vi "Migrate InstrumentStudio Plug-in.vi"() -> ()   [LabVIEW 2021]
uses:
  _Measurement Migrator/Migrator/Queue Driver/controls/Queue Operations.ctl
  _Measurement Migrator/Migrator/Migration Logic/controls/Multiple Migration/Multiple Migration Data Holder.ctl
  <vilib>/Utility/sysdir.llb/System Directory Type.ctl
  <vilib>/Utility/miscctls.llb/LVRowAndColumnUnsignedTypeDef.ctl
  <vilib>/Utility/miscctls.llb/LVRowAndColumnTypeDef.ctl
  _Measurement Migrator/Migrator/Migrator Reusables/controls/Dictionary States.ctl
  <vilib>/Utility/cursorutil.llb/Set Cursor (Icon Pict).vi
  _Measurement Migrator/Migrator/Queue Driver/Queue Driver.lvlib
  _Measurement Migrator/Migrator/Migration Logic/Migrator.lvlib
  _Measurement Migrator/Migrator/Path Functions/Path Functions.lvlib
  _Measurement Migrator/Migrator/Multiple Migrator/Multiple Migrator.lvlib
  _Measurement Migrator/Migrator/Migrator Reusables/Migrator Reusables.lvlib
  _Measurement Migrator/Migrator/G Plug-in Migrator/G Plug-in Migrator.lvlib
panel:
  out "error out":errorcluster
  in  "Tab Control":T1(tab)
  in  "Info":string
  in  "Select Measurement":path
  out "Warning":bool=TRUE caption="Warning:\nSelected folder contains invalid folder/file names"
  in  "Populate measurements":bool
  in  "Select Project":path
  in  "Select all":bool
  in  "Back to Home":bool
  in  "List Plug-ins":bool
  in  "Select Measurements":string(tree)
  out "Selection warning":string="Atleast one measurement should be selected"
  out "Plug-in info":string="* Rename the Plug-in if required"
  out "Plug-in warning":string="Warning:\n1. Measurement plug-in name must be unique \n2. Plugin name cannot contain any of the following characters:\n         \\ / : * ? \" < > |"
  in  "Start Migration":bool
  in  "Back to Select":bool
  in  "List of Selected Measurements":i32(listbox)
  in  "Measurement Count":i32(slide)=6 caption="Migrating 2 of 2 measurement(s)" scale=0.0..100.0
  in  "Progress":i32(slide)=9 caption="Saving the project files..." scale=0.0..15.0
  in  "Review":bool
  in  "Migration Status":i32(listbox)
  in  "Back to Status":bool
  in  "Select Plug-in":string(combo) caption="Select G plug-in to review"
  in  "Start Next":bool
  out "Launch Gplugin":string
  out "Launch VI":string
  # "* Project in which the measurement plug-in will be created"
  # "* Select a measurement vi or a folder containing measurements"
  # ".lvproj"
  # "Select the measurements to migrate"
  # "Review the G Plug-in:\n1. Review the Main VI. Click here to launch.\n2. Review the G plug-in data file. Click here to launch."
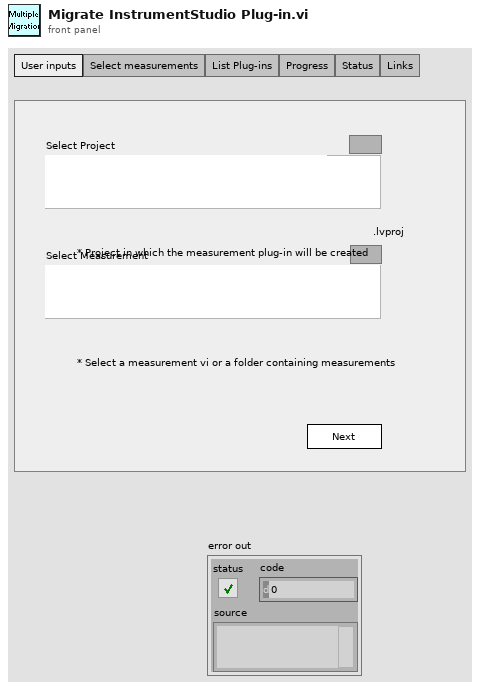
[diagram p1: front panel]
types:
  T1 = enum32{"User inputs", "Select measurements", "List Plug-ins", "Progress", "Status", "Links"}
  T2 = typedef "Queue Driver.lvlib/Queue Operations.ctl" = enum16{"Create Q", "Enqueue", "Enqueue N", "Dequeue", "Flush", "Release"}
  T3 = typedef "Migrator.lvlib/Multiple Migration Data Holder.ctl" = cluster{"Tree Reference":refnum<vi>, "LabVIEW Version":string, "Project path":path, "Create new project?":bool, "Measurement file/folder path":path, "Measurement folder selected?":bool, "Project warning":string, "Measurement warning":string, "Next clicked?":bool, "Measurement path changed?":bool, "Select all":bool, "Measurement folder Tags":string[], "Measurement file Tags":string[], "Selected cell Tag":string, "Measurement Plug-ins":string[][], "Measurement File Paths":path[], "Plugin Migration Value":i32, "Migration Count":i32, "Instrument containing subVIs":path[][], "Progress per measurement":i32, "Measurement Progress":i32, "Migration Status":string[][], "Selected Measurement":string[], "G plugin Path":path[], "Plugin data file":path[], "Index":i32}
  T4 = enum8{"Enabled", "Disabled", "Disabled and Grayed Out"}
  T5 = typedef "LVRowAndColumnUnsignedTypeDef.ctl" = cluster{"Row":u32, "Column":u32}
  T6 = typedef "LVRowAndColumnTypeDef.ctl" = cluster{"Row":i32, "Column":i32}
  T7 = typedef "Migrator Reusables.lvlib/Dictionary States.ctl" = enum16{"Set", "Get", "Delete", "Delete All"}
  T8 = typedef "System Directory Type.ctl" = i32
  T9 = typedef "LVPoint32TypeDef.ctl" = cluster{"Horizontal":i32, "Vertical":i32}
  T10 = typedef "Migrator.lvlib/Tree Items.ctl" = cluster{"Item name":string, "Indent":i32, "Tag":string}
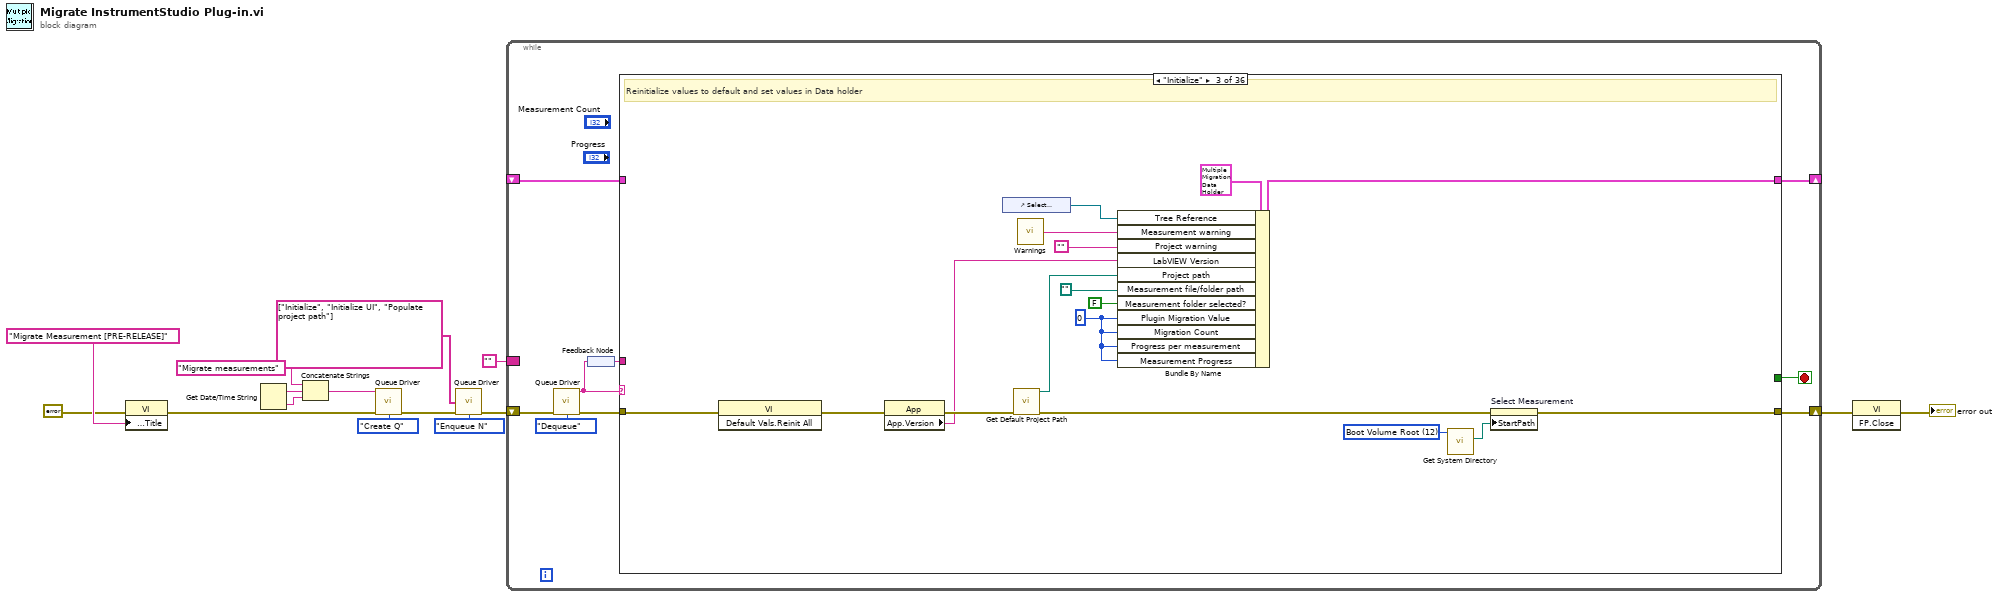
[diagram p0: block diagram]
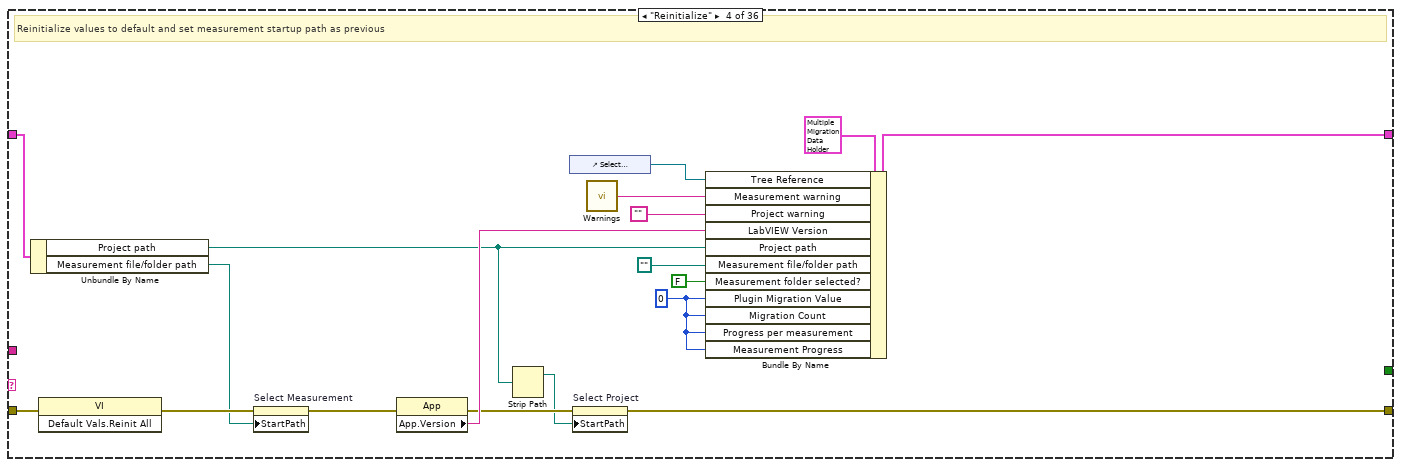
[diagram p4: hidden frame]
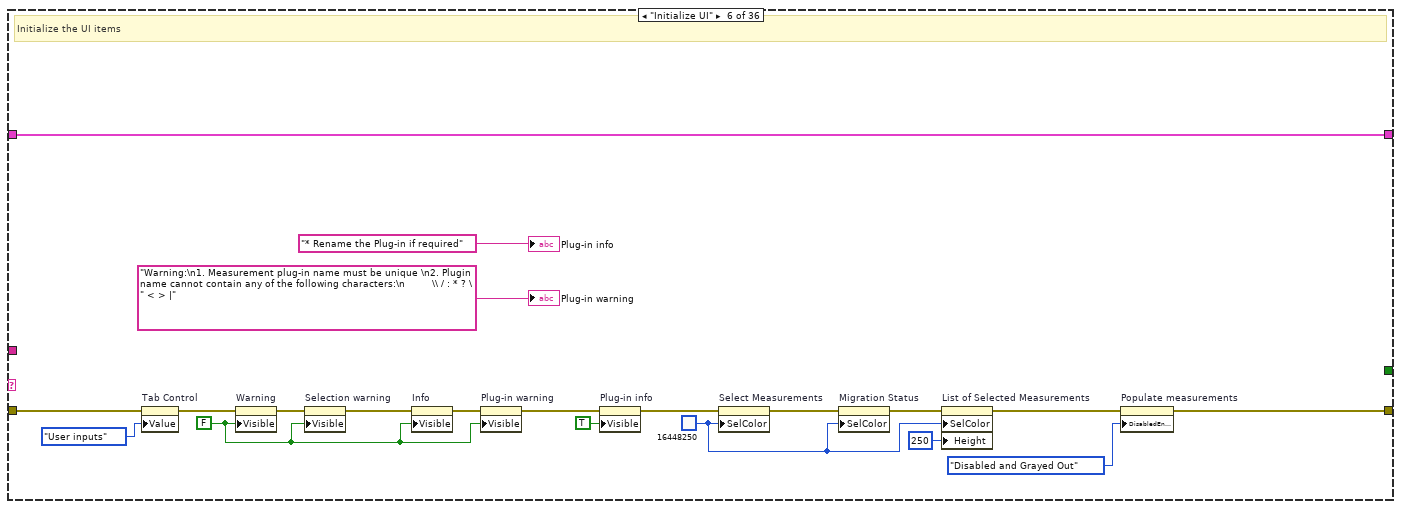
[diagram p6: hidden frame]
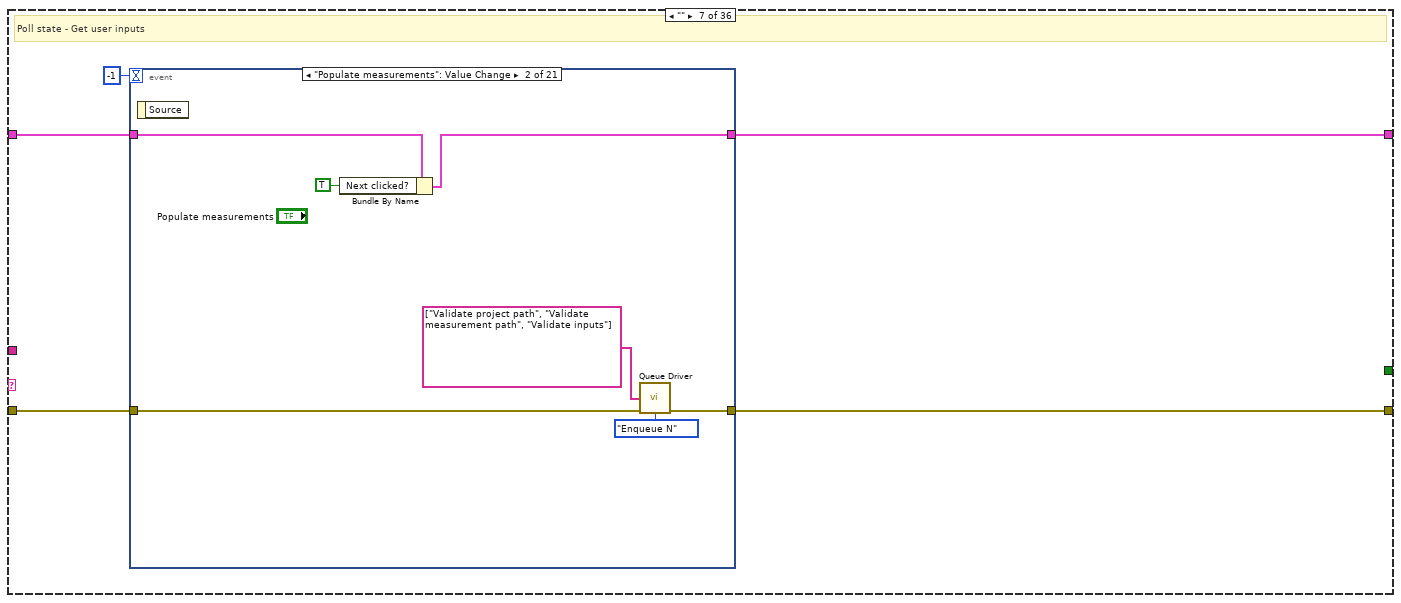
[diagram p7: hidden frame]
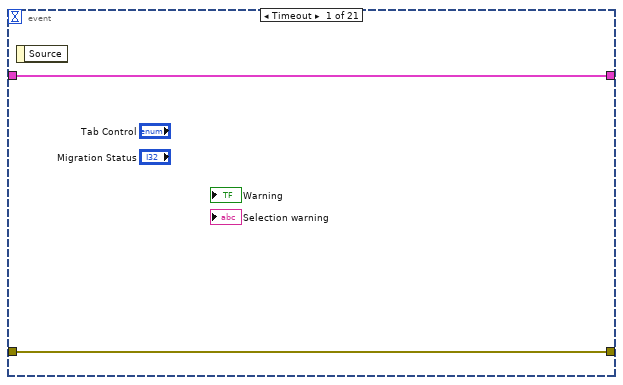
[diagram p8: hidden frame]
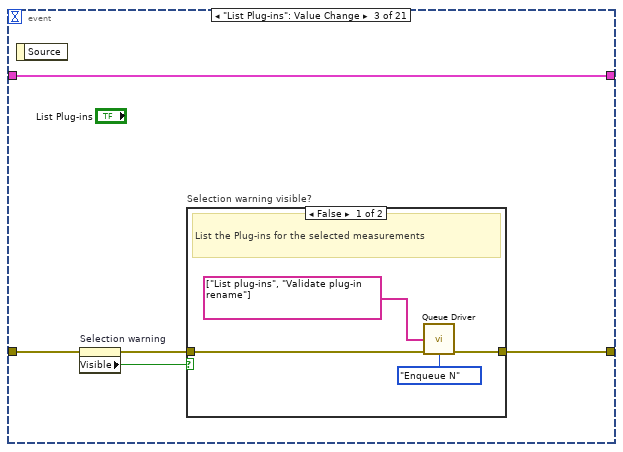
[diagram p9: hidden frame]
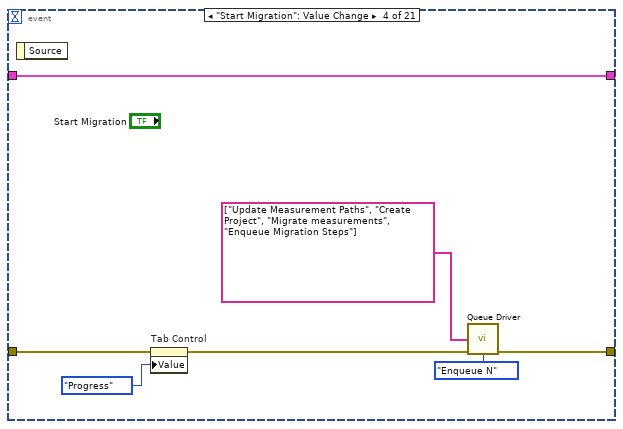
[diagram p11: hidden frame]
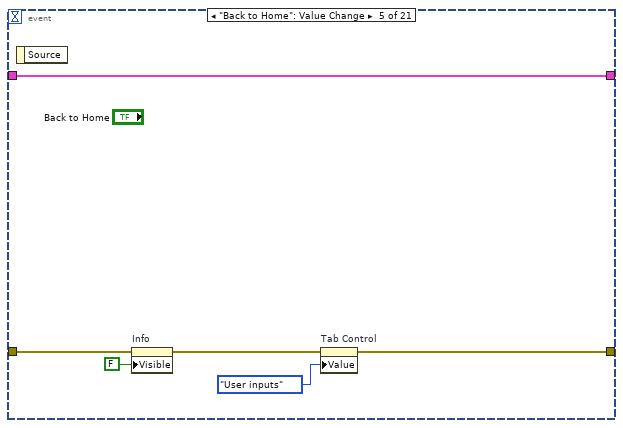
[diagram p12: hidden frame]
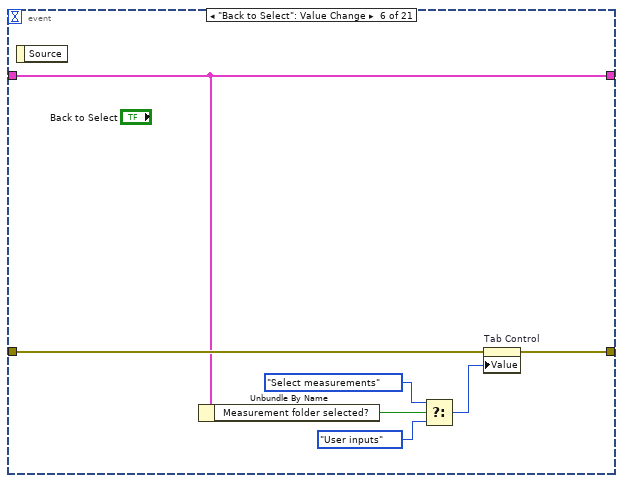
[diagram p13: hidden frame]
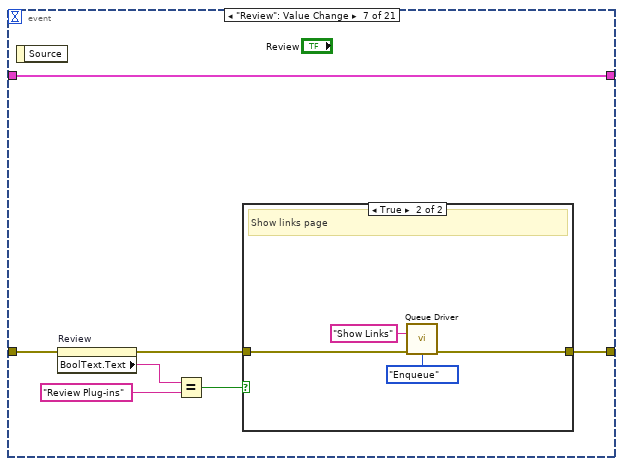
[diagram p14: hidden frame]
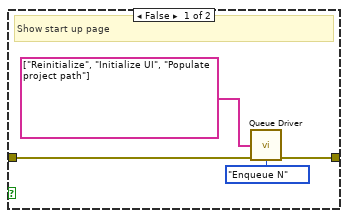
[diagram p15: hidden frame]
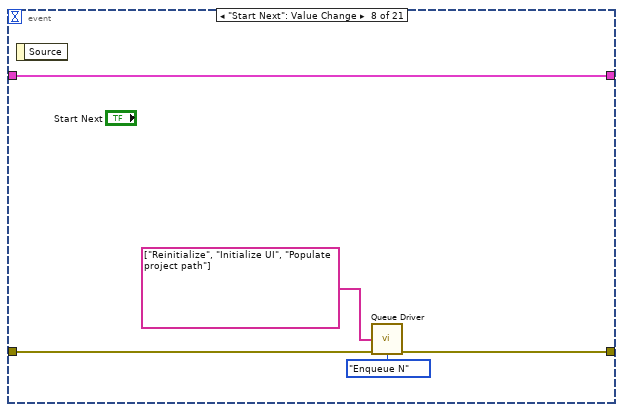
[diagram p16: hidden frame]
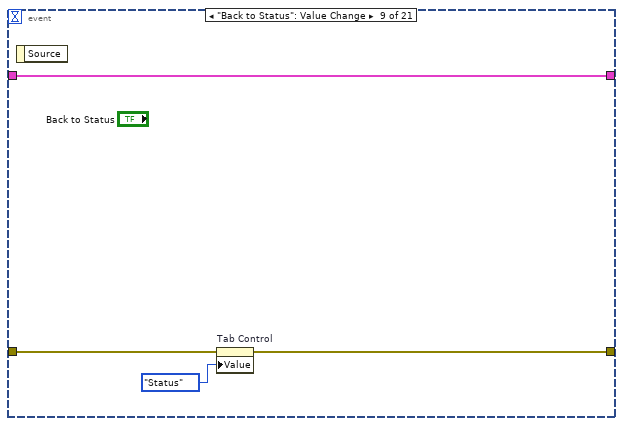
[diagram p17: hidden frame]
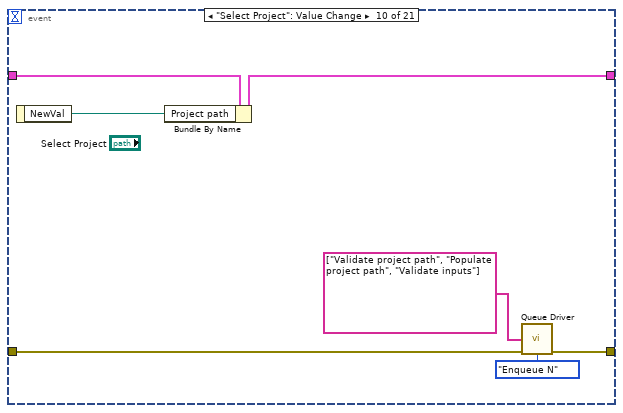
[diagram p18: hidden frame]
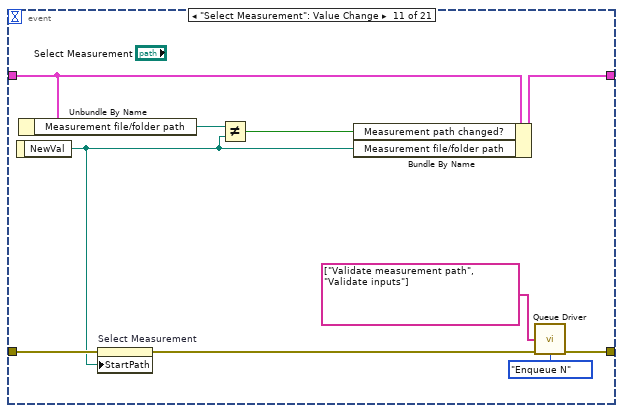
[diagram p19: hidden frame]
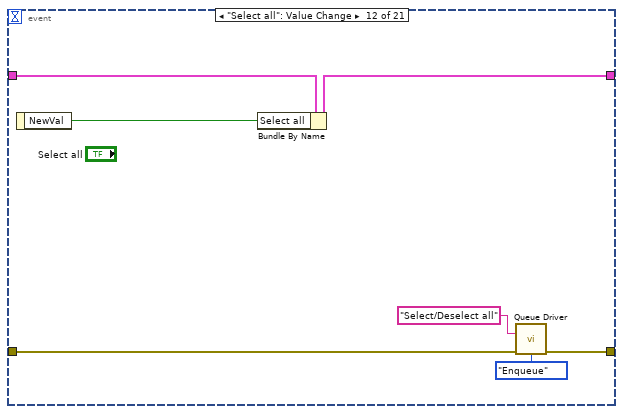
[diagram p20: hidden frame]
diagram:
  n1 = property class="VI"(error in=errorcluster {"status"=FALSE, "code"=0, "source"=""} ("error in (no error)"), "Front Panel.Title"="Migrate Measurement [PRE-RELEASE]" ("Front Panel Window:Title")) -> (error out=w1:errorcluster)  [unwired: 1 in, 1 out]
  n2 = Get Date/Time String() -> (date string=w12:string, time string=w11:string)  [unwired: 3 in]
  n3 = Concatenate Strings("Migrate measurements" ("string"), w12, w11) -> (w7:string)
  n4 = call "Queue Driver.vi"("Name"=w7, "error in (no error)"=w1, "Q Operations"=Queue_Operations."Create Q") -> ("error out"=w15:errorcluster)  [unwired: 11 in, 1 out]
  n5 = call "Queue Driver.vi"("States[]"=string[] ["Initialize", "Initialize UI", "Populate project path"], "error in (no error)"=w15, "Q Operations"=Queue_Operations."Enqueue N") -> ("error out"=w10:errorcluster)  [unwired: 11 in, 1 out]
  n6 = while {
    shift-right: [w23] -> w6
    shift-left: w10 -> [w24]
    shift-right: [w20] -> _
    shift-left: _ -> [w19]
    border: "" -> [_]
    stop <- w18 stop-if-true
    n7 = call "Queue Driver.vi"("error in (no error)"=w24, "Q Operations"=Queue_Operations."Dequeue") -> ("Dequeued State"=w17:string, "error out"=w22:errorcluster)  [unwired: 12 in]
    n8 = feedback #1() -> (w16:string)
    n9 = feedback-in #1(w17) -> ()
    n10 = case shown="\"Initialize\"" w17 {
      tunnel: w22 -> [w25 w28 w45 w63 w65 w85 w90 w258 w270 w281 w300 w324 w369 w386 w439 w464 w485 w511 w547 w557 w564 w584 w594 w613 w630 w664 w673 w679 w701 w722 w734 w777 w786 w795 w816 w828]
      tunnel: [w25 w28 w34 w48 w65 w76 w89 w260 w270 w273 w299 w323 w369 w381 w427 w447 w472 w510 w537 w557 w559 w581 w597 w612 w629 w650 w674 w683 w705 w722 w733 w774 w786 w792 w816 w818] -> w23
      tunnel: [w26 w27 w44 w62 w64 w81 w86 w259 w271 w276 w293 w311 w370 w387 w430 w462 w469 w508 w542 w556 w576 w592 w606 w616 w649 w651 w677 w684 w706 w723 w738 w769 w787 w797 w817 w826] -> w20
      tunnel: w19 -> [w26 w27 _ w51 w64 w81 w87 w259 w271 w277 w295 w322 w370 w388 w431 w463 w470 w509 w543 w556 w577 w592 w605 w616 w649 w653 w677 w685 w707 w723 w739 w776 w787 w797 w817 w826]
      tunnel: [_ _ _ _ _ _ _ _ _ _ _ _ _ _ _ _ _ _ _ _ _ _ _ _ _ _ _ _ _ _ _ _ _ _ _ TRUE] -> w18
      tunnel: w16 -> [_ _ _ _ _ _ _ _ _ _ _ _ _ _ _ _ _ _ _ _ _ _ _ _ _ _ _ _ _ _ _ _ _ w788 _ _]
      frame Default {
        # "Default case"
      }
      frame "/**********INITIALIZE**********/" {
      }
      frame "Initialize" {
        w29 = 0 ("Plugin Migration Value")
        w33 = T8 12 items=["User Home"=0, "User Desktop"=1, "User Documents"=2, "User Application Data"=3, "User Preferences"=4, "User Temporary"=5, "Public Documents"=6, "Public Application Data"=7, "Public Preferences"=8, "Public Cache"=13, "System Core Libraries"=9, "System Installed Libraries"=10, "Application Files"=11, "Boot Volume Root"=12] ("system directory type")
        # "Reinitialize values to default and set values in Data holder"
        n11 = invoke class="VI" method="Default Vals.Reinit All"(error in=w45) -> (error out=w42:errorcluster)  [unwired: 2 in, 2 out]
        n12 = property class="App"(error in=w42) -> (error out=w41:errorcluster, "App.Version"=w40:string)  [unwired: 1 in, 1 out]
        n13 = control-ref of="Select Measurements"() -> (w37:refnum<vi>)
        n14 = call "Get Default Project Path.vi"("error in"=w41) -> ("Project Path"=w43:path, "error out"=w35:errorcluster)  [unwired: 13 in]
        n15 = call "Warnings.vi"() -> ("Invalid measurement path"=w36:string)  [unwired: 8 in, 7 out]
        n16 = Bundle By Name(cluster=T3 {"Tree Reference"=refnum, "LabVIEW Version"="", "Project path"=path "", "Create new project?"=FALSE, "Measurement file/folder path"=path "", "Measurement folder selected?"=FALSE, "Project warning"="", "Measurement warning"="", "Next clicked?"=FALSE, "Measurement path changed?"=FALSE, "Select all"=FALSE, "Measurement folder Tags"=[], "Measurement file Tags"=[], "Selected cell Tag"="", "Measurement Plug-ins"=[], "Measurement File Paths"=[], "Plugin Migration Value"=0, "Migration Count"=0, "Instrument containing subVIs"=[], "Progress per measurement"=0, "Measurement Progress"=0, "Migration Status"=[], "Selected Measurement"=[], "G plugin Path"=[], "Plugin data file"=[], "Index"=0}, "Tree Reference"=w37, "Measurement warning"=w36, "Project warning"="", "LabVIEW Version"=w40, "Project path"=w43, "Measurement file/folder path"=path "", "Measurement folder selected?"=FALSE, "Plugin Migration Value"=w29, "Migration Count"=w29, "Progress per measurement"=w29, "Measurement Progress"=w29) -> (w44:T3)
        n17 = call <vilib>:"Get System Directory.vi"("system directory type"=w33) -> ("system directory"=w32:path)  [unwired: 10 in]
        n18 = property on="Select Measurement" class="Path"(error in=w35, "StartPath"=w32) -> (error out=w34:errorcluster)  [unwired: 1 in, 1 out]
      }
      frame "Reinitialize" {
        w54 = 0 ("Plugin Migration Value")
        # "Reinitialize values to default and set measurement startup path as previous"
        n19 = Unbundle By Name(w51) -> ("Project path"=w47:path, "Measurement file/folder path"=w50:path)
        n20 = invoke class="VI" method="Default Vals.Reinit All"(error in=w63) -> (error out=w53:errorcluster)  [unwired: 2 in, 2 out]
        n21 = property on="Select Measurement" class="Path"(error in=w53, "StartPath"=w50) -> (error out=w52:errorcluster)  [unwired: 1 in, 1 out]
        n22 = property class="App"(error in=w52) -> (error out=w49:errorcluster, "App.Version"=w61:string)  [unwired: 1 in, 1 out]
        n23 = Strip Path(path=w47) -> (stripped path=w46:path)  [unwired: 1 out]
        n24 = control-ref of="Select Measurements"() -> (w58:refnum<vi>)
        n25 = property on="Select Project" class="Path"(error in=w49, "StartPath"=w46) -> (error out=w48:errorcluster)  [unwired: 1 in, 1 out]
        n26 = call "Warnings.vi"() -> ("Invalid measurement path"=w57:string)  [unwired: 8 in, 7 out]
        n27 = Bundle By Name(cluster=T3 {"Tree Reference"=refnum, "LabVIEW Version"="", "Project path"=path "", "Create new project?"=FALSE, "Measurement file/folder path"=path "", "Measurement folder selected?"=FALSE, "Project warning"="", "Measurement warning"="", "Next clicked?"=FALSE, "Measurement path changed?"=FALSE, "Select all"=FALSE, "Measurement folder Tags"=[], "Measurement file Tags"=[], "Selected cell Tag"="", "Measurement Plug-ins"=[], "Measurement File Paths"=[], "Plugin Migration Value"=0, "Migration Count"=0, "Instrument containing subVIs"=[], "Progress per measurement"=0, "Measurement Progress"=0, "Migration Status"=[], "Selected Measurement"=[], "G plugin Path"=[], "Plugin data file"=[], "Index"=0}, "Tree Reference"=w58, "Measurement warning"=w57, "Project warning"="", "LabVIEW Version"=w61, "Project path"=w47, "Measurement file/folder path"=path "", "Measurement folder selected?"=FALSE, "Plugin Migration Value"=w54, "Migration Count"=w54, "Progress per measurement"=w54, "Measurement Progress"=w54) -> (w62:T3)
      }
      frame "/**********FP RELATED**********/" {
      }
      frame "Initialize UI" {
        w70 = FALSE ("Visible")
        w78 = u32 16448250 ("Selection Color")
        # "Initialize the UI items"
        n28 = property on="Tab Control" class="TabCtl (strict)"(error in=w85, "Value"=T1."User inputs" ("Tab Control")) -> (error out=w80:errorcluster)  [unwired: 1 in, 1 out]
        n29 = property on="Warning" class="Bool"(error in=w80, "Visible"=w70) -> (error out=w79:errorcluster)  [unwired: 1 in, 1 out]
        n30 = property on="Selection warning" class="Str"(error in=w79, "Visible"=w70) -> (error out=w74:errorcluster)  [unwired: 1 in, 1 out]
        n31 = property on="Info" class="Str"(error in=w74, "Visible"=w70) -> (error out=w73:errorcluster)  [unwired: 1 in, 1 out]
        n32 = property on="Plug-in warning" class="Str"(error in=w73, "Visible"=w70) -> (error out=w69:errorcluster)  [unwired: 1 in, 1 out]
        n33 = property on="Plug-in info" class="Str"(error in=w69, "Visible"=TRUE) -> (error out=w68:errorcluster)  [unwired: 1 in, 1 out]
        n34 = property on="Select Measurements" class="Tree (strict)"(error in=w68, "SelColor"=w78) -> (error out=w83:errorcluster)  [unwired: 1 in, 1 out]
        n35 = property on="Migration Status" class="MCListbox (strict)"(error in=w83, "SelColor"=w78) -> (error out=w82:errorcluster)  [unwired: 1 in, 1 out]
        n36 = property on="List of Selected Measurements" class="MCListbox (strict)"(error in=w82, "SelColor"=w78, "Height"=u32 250 ("Size:Height")) -> (error out=w77:errorcluster)  [unwired: 1 in, 1 out]
        n37 = property on="Populate measurements" class="Bool"(error in=w77, "DisabledEnum"=T4."Disabled and Grayed Out" ("Disabled")) -> (error out=w76:errorcluster)  [unwired: 1 in, 1 out]
        "Plug-in warning" <- "Warning:\n1. Measurement plug-in name must be unique \n2. Plugin name cannot contain any of the following characters:\n         \\ / : * ? \" < > |" ("f")
        "Plug-in info" <- "* Rename the Plug-in if required" ("Plug-in warning")
      }
      frame "" {
        # "Poll state - Get user inputs"
        n38 = event shown="[1] \"Populate measurements\": Value Change" {
          selector: _ -> [_ _ _ _ _ _ _ _ _ _ _ _ _ _ _ _ _ _ _ _ _]
          dyn-events: _ -> [_ _ _ _ _ _ _ _ _ _ _ _ _ _ _ _ _ _ _ _ _]
          timeout: -1 -> [_ _ _ _ _ _ _ _ _ _ _ _ _ _ _ _ _ _ _ _ _]
          tunnel: w90 -> [w92 w99 w102 w116 w119 w129 w133 w146 w153 w160 w166 w174 w185 w194 w202 w213 w215 w219 w226 w238 w252]
          tunnel: [w92 w98 w103 w112 w122 w128 w135 w147 w152 w159 w169 w173 w180 w193 w200 w212 w216 w220 w228 w241 w251] -> w89
          tunnel: w87 -> [w91 w95 w104 w113 w120 w127 w136 w149 w150 w157 w164 w177 w184 w195 w203 w214 w218 w222 w223 w236 w253]
          tunnel: [w91 w94 w104 w113 w120 w127 w136 w149 w150 w156 w170 w176 w183 w195 w203 w209 w218 w222 w223 w236 w253] -> w86
          event Timeout {
            # "Timeout"
            n39 = event-data() -> ()  [unwired: 1 in, 1 out]
          }
          event "Populate measurements": Value Change {
            n40 = event-data() -> ()  [unwired: 1 in, 1 out]
            n41 = Bundle By Name(cluster=w95, "Next clicked?"=TRUE) -> (w94:T3)
            n42 = call "Queue Driver.vi"("States[]"=string[] ["Validate project path", "Validate measurement path", "Validate inputs"], "error in (no error)"=w99, "Q Operations"=Queue_Operations."Enqueue N") -> ("error out"=w98:errorcluster)  [unwired: 11 in, 1 out]
          }
          event "List Plug-ins": Value Change {
            n43 = event-data() -> ()  [unwired: 1 in, 1 out]
            n44 = property on="Selection warning" class="Str"(error in=w102) -> (error out=w101:errorcluster, "Visible"=w100:bool)  [unwired: 1 in, 1 out]
            n45 = case "Selection warning visible?" shown="False" w100 {
              tunnel: w101 -> [w108 w109]
              tunnel: [w107 w109] -> w103
              frame False {
                # "List the Plug-ins for the selected measurements"
                n46 = call "Queue Driver.vi"("States[]"=string[] ["List plug-ins", "Validate plug-in rename"], "error in (no error)"=w108, "Q Operations"=Queue_Operations."Enqueue N") -> ("error out"=w107:errorcluster)  [unwired: 11 in, 1 out]
              }
              frame True {
                # "Pass"
              }
            }
          }
          event "Start Migration": Value Change {
            n47 = event-data() -> ()  [unwired: 1 in, 1 out]
            n48 = property on="Tab Control" class="TabCtl (strict)"(error in=w116, "Value"=T1."Progress" ("Tab Control")) -> (error out=w115:errorcluster)  [unwired: 1 in, 1 out]
            n49 = call "Queue Driver.vi"("States[]"=string[] ["Update Measurement Paths", "Create Project", "Migrate measurements", "Enqueue Migration Steps"], "error in (no error)"=w115, "Q Operations"=Queue_Operations."Enqueue N") -> ("error out"=w112:errorcluster)  [unwired: 11 in, 1 out]
          }
          event "Back to Home": Value Change {
            n50 = event-data() -> ()  [unwired: 1 in, 1 out]
            n51 = property on="Info" class="Str"(error in=w119, "Visible"=FALSE) -> (error out=w118:errorcluster)  [unwired: 1 in, 1 out]
            n52 = property on="Tab Control" class="TabCtl (strict)"(error in=w118, "Value"=T1."User inputs" ("Tab Control")) -> (error out=w122:errorcluster)  [unwired: 1 in, 1 out]
          }
          event "Back to Select": Value Change {
            n53 = event-data() -> ()  [unwired: 1 in, 1 out]
            n54 = Unbundle By Name(w127) -> ("Measurement folder selected?"=w126:bool)
            n55 = Select(t=T1."Select measurements" ("Tab Control"), s=w126, f=T1."User inputs" ("Tab Control")) -> (s? t:f=w123:T1)
            n56 = property on="Tab Control" class="TabCtl (strict)"(error in=w129, "Value"=w123) -> (error out=w128:errorcluster)  [unwired: 1 in, 1 out]
          }
          event "Review": Value Change {
            n57 = event-data() -> ()  [unwired: 1 in, 1 out]
            n58 = property on="Review" class="Bool"(error in=w133) -> (error out=w134:errorcluster, "BoolText.Text"=w132:string)  [unwired: 1 in, 1 out]
            n59 = Equal?(x=w132, y="Review Plug-ins") -> (x = y?=w130:bool)
            n60 = case shown="True" w130 {
              tunnel: [w138 w144] -> w135
              tunnel: w134 -> [w137 w141]
              frame False {
                # "Show start up page"
                n61 = call "Queue Driver.vi"("States[]"=string[] ["Reinitialize", "Initialize UI", "Populate project path"], "error in (no error)"=w137, "Q Operations"=Queue_Operations."Enqueue N") -> ("error out"=w138:errorcluster)  [unwired: 11 in, 1 out]
              }
              frame True {
                # "Show links page"
                n62 = call "Queue Driver.vi"("State"="Show Links", "error in (no error)"=w141, "Q Operations"=Queue_Operations."Enqueue") -> ("error out"=w144:errorcluster)  [unwired: 11 in, 1 out]
              }
            }
          }
          event "Start Next": Value Change {
            n63 = event-data() -> ()  [unwired: 1 in, 1 out]
            n64 = call "Queue Driver.vi"("States[]"=string[] ["Reinitialize", "Initialize UI", "Populate project path"], "error in (no error)"=w146, "Q Operations"=Queue_Operations."Enqueue N") -> ("error out"=w147:errorcluster)  [unwired: 11 in, 1 out]
          }
          event "Back to Status": Value Change {
            n65 = event-data() -> ()  [unwired: 1 in, 1 out]
            n66 = property on="Tab Control" class="TabCtl (strict)"(error in=w153, "Value"=T1."Status" ("Tab Control")) -> (error out=w152:errorcluster)  [unwired: 1 in, 1 out]
          }
          event "Select Project": Value Change {
            n67 = event-data() -> ("NewVal"=w155:path)  [unwired: 1 in]
            n68 = Bundle By Name(cluster=w157, "Project path"=w155) -> (w156:T3)
            n69 = call "Queue Driver.vi"("States[]"=string[] ["Validate project path", "Populate project path", "Validate inputs"], "error in (no error)"=w160, "Q Operations"=Queue_Operations."Enqueue N") -> ("error out"=w159:errorcluster)  [unwired: 11 in, 1 out]
          }
          event "Select Measurement": Value Change {
            n70 = event-data() -> ("NewVal"=w161:path)  [unwired: 1 in]
            n71 = Unbundle By Name(w164) -> ("Measurement file/folder path"=w162:path)
            n72 = property on="Select Measurement" class="Path"(error in=w166, "StartPath"=w161) -> (error out=w165:errorcluster)  [unwired: 1 in, 1 out]
            n73 = Not Equal?(x=w162, y=w161) -> (x != y?=w163:bool)
            n74 = Bundle By Name(cluster=w164, "Measurement path changed?"=w163, "Measurement file/folder path"=w161) -> (w170:T3)
            n75 = call "Queue Driver.vi"("States[]"=string[] ["Validate measurement path", "Validate inputs"], "error in (no error)"=w165, "Q Operations"=Queue_Operations."Enqueue N") -> ("error out"=w169:errorcluster)  [unwired: 11 in, 1 out]
          }
          event "Select all": Value Change {
            n76 = event-data() -> ("NewVal"=w175:bool)  [unwired: 1 in]
            n77 = Bundle By Name(cluster=w177, "Select all"=w175) -> (w176:T3)
            n78 = call "Queue Driver.vi"("State"="Select/Deselect all", "error in (no error)"=w174, "Q Operations"=Queue_Operations."Enqueue") -> ("error out"=w173:errorcluster)  [unwired: 11 in, 1 out]
          }
          event "Select Measurements": Mouse Down {
            n79 = event-data() -> ("Coords"=w178:T9)  [unwired: 1 in]
            n80 = invoke on="Select Measurements" class="Tree (strict)" method="Point To Row Column"(error in=w185, "Point"=w178) -> (error out=w181:errorcluster, "Tag"=w182:string, "InGlyph"=w179:bool)  [unwired: 6 in, 5 out]
            n81 = case "In Symbol?" shown="True" w179 {
              tunnel: w181 -> [w186 w190]
              tunnel: [w186 w189] -> w180
              frame False {
                # "Pass"
              }
              frame True {
                # "Update the selection of measurements"
                n82 = call "Queue Driver.vi"("State"="Measurement selection" ("State 2"), "error in (no error)"=w190, "Q Operations"=Queue_Operations."Enqueue") -> ("error out"=w189:errorcluster)  [unwired: 11 in, 1 out]
              }
            }
            n83 = Bundle By Name(cluster=w184, "Selected cell Tag"=w182) -> (w183:T3)
          }
          event "List of Selected Measurements": Edit Cell {
            n84 = event-data() -> ()  [unwired: 1 in, 1 out]
            n85 = call "Queue Driver.vi"("State"="Update plugin name", "error in (no error)"=w194, "Q Operations"=Queue_Operations."Enqueue") -> ("error out"=w193:errorcluster)  [unwired: 11 in, 1 out]
          }
          event "List of Selected Measurements": Mouse Down {
            n86 = event-data() -> ("Coords"=w199:T9)  [unwired: 1 in, 7 out]
            n87 = invoke on="List of Selected Measurements" class="MCListbox (strict)" method="Point To Row Column"(error in=w202, "Point"=w199) -> (error out=w201:errorcluster, "CellPosition"=w196:T6)  [unwired: 5 in, 5 out]
            n88 = Unbundle By Name(w196) -> ("Column"=w198:i32)
            n89 = Not Equal To 0?(x=w198) -> (x != 0?=w197:bool)
            n90 = case shown="True" w197 {
              tunnel: w201 -> [w204 w207]
              tunnel: [w204 w206] -> w200
              tunnel: w196 -> [_ w205]
              frame False {
              }
              frame True {
                n91 = property on="List of Selected Measurements" class="MCListbox (strict)"(error in=w207, "EditPos"=w205) -> (error out=w206:errorcluster)  [unwired: 1 in, 1 out]
              }
            }
          }
          event "Select Plug-in": Value Change {
            n92 = event-data() -> ("NewVal"=w210:string)  [unwired: 1 in]
            n93 = property on="Select Plug-in" class="CmbBox"(error in=w213) -> (error out=w212:errorcluster, "Strings[]"=w211:string[])  [unwired: 1 in, 1 out]
            n94 = Search 1D Array(1D array=w211, element=w210) -> (index of element=w208:i32)  [unwired: 1 in]
            n95 = Bundle By Name(cluster=w214, "Index"=w208) -> (w209:T3)
          }
          event "Launch VI", "Launch Gplugin": Mouse Enter {
            n96 = event-data() -> ()  [unwired: 1 in, 1 out]
            n97 = call-poly <vilib>:"Set Cursor.vi"("error in (no error)"=w215, "icon"=u16 6) -> ("error out"=w216:errorcluster)  [unwired: 8 in, 1 out]
          }
          event "Launch VI", "Launch Gplugin": Mouse Leave {
            n98 = event-data() -> ()  [unwired: 1 in, 1 out]
            n99 = call-poly <vilib>:"Set Cursor.vi"("error in (no error)"=w219, "icon"=u16 0) -> ("error out"=w220:errorcluster)  [unwired: 8 in, 1 out]
          }
          event "Launch VI": Mouse Down {
            n100 = event-data() -> ()  [unwired: 1 in, 1 out]
            n101 = property on="Select Plug-in" class="CmbBox"(error in=w226) -> (error out=w227:errorcluster, "Value"=w225:string)  [unwired: 1 in, 1 out]
            n102 = Empty String/Path?(string/path=w225) -> (empty?=w224:bool)
            n103 = case shown="False" w224 {
              tunnel: [w234 w235] -> w228
              tunnel: w227 -> [w233 w235]
              tunnel: w223 -> [w232 _]
              frame False {
                n104 = Unbundle By Name(w232) -> ("G plugin Path"=w231:path[], "Index"=w230:i32)
                n105 = Index Array(array=w231, index=w230) -> (element=w229:path)
                n106 = call "Open VI.vi"("Logic VI Path"=w229, "error in (no error)"=w233) -> ("error out"=w234:errorcluster)  [unwired: 13 in]
              }
              frame True {
              }
            }
          }
          event "Launch Gplugin": Mouse Down {
            n107 = event-data() -> ()  [unwired: 1 in, 1 out]
            n108 = property on="Select Plug-in" class="CmbBox"(error in=w238) -> (error out=w239:errorcluster, "Value"=w240:string)  [unwired: 1 in, 1 out]
            n109 = Empty String/Path?(string/path=w240) -> (empty?=w237:bool)
            n110 = case shown="False" w237 {
              tunnel: [w243 w248] -> w241
              tunnel: w239 -> [w242 w248]
              tunnel: w236 -> [w245 _]
              frame False {
                n111 = Unbundle By Name(w245) -> ("Plugin data file"=w247:path[], "Index"=w246:i32)
                n112 = Index Array(array=w247, index=w246) -> (element=w244:path)
                n113 = call "Open plugin data.vi"("Path"=w244, "error in (no error)"=w242) -> ("error out"=w243:errorcluster)  [unwired: 13 in]
              }
              frame True {
              }
            }
          }
          event Panel Close? {
            n114 = event-data() -> ()  [unwired: 1 in, 1 out]
            n115 = call "Queue Driver.vi"("State"="Exit", "error in (no error)"=w252, "Q Operations"=Queue_Operations."Enqueue") -> ("error out"=w251:errorcluster)  [unwired: 11 in, 1 out]
            n116 = event-data("Discard?"=TRUE) -> ()  [unwired: 1 in, 1 out]
          }
        }
      }
      frame "Populate project path" {
        # "Populate the validated project path in the control"
        n117 = Unbundle By Name(w259) -> ("Project warning"=w256:string, "Project path"=w257:path)
        n118 = Empty String/Path?(string/path=w256) -> (empty?=w255:bool)
        n119 = case "Valid project?" shown="True" w255 {
          tunnel: [w261 w269] -> w260
          tunnel: w258 -> [w261 w268]
          tunnel: w257 -> [_ w263]
          frame False {
            # "Pass"
          }
          frame True {
            # "Populate the path in the control"
            n120 = call <vilib>:"Get File Extension.vi"("error in (no error)"=w268, "file"=w263) -> ("error out"=w267:errorcluster, "filename without extension"=w266:string)  [unwired: 5 in, 3 out]
            n121 = Concatenate Strings("..\\" ("string"), w266) -> (w264:string)
            n122 = Build Path(base path=w263, name or relative path=w264) -> (appended path=w262:path)
            n123 = property on="Select Project" class="Path"(error in=w267, "Value"=w262) -> (error out=w269:errorcluster)  [unwired: 1 in, 1 out]
          }
        }
      }
      frame "/**********INPUT VALIDATION**********/" {
      }
      frame "Validate project path" {
        # "Validate the project path and set warning if required"
        n124 = Unbundle By Name(w277) -> ("Project path"=w278:path, "LabVIEW Version"=w279:string)
        n125 = call <vilib>:"Is Path and Not Empty.vi"("path"=w278) -> ("Is Path and Not Empty?"=w280:bool)  [unwired: 4 in]
        n126 = case "Is Path and not empty?" shown="True" w280 {
          tunnel: w281 -> [w284 w291]
          tunnel: [w284 w290] -> w273
          tunnel: [w282 w289] -> w272
          tunnel: w279 -> [_ w288]
          tunnel: w278 -> [w283 w287]
          tunnel: [_ w286] -> w275
          tunnel: [w283 w285] -> w274
          frame False {
            # "Set warning"
            n127 = call "Warnings.vi"() -> ("Invalid project path"=w282:string)  [unwired: 8 in, 7 out]
          }
          frame True {
            # "Validate the path"
            n128 = call "Validate Project Path.vi"("Project path in"=w287, "LabVIEW Version"=w288, "error in (no error)"=w291) -> ("Validated project path"=w285:path, "New project?"=w286:bool, "Warning"=w289:string, "error out"=w290:errorcluster)  [unwired: 9 in]
          }
        }
        n129 = Bundle By Name(cluster=w277, "Project path"=w274, "Create new project?"=w275, "Project warning"=w272) -> (w276:T3)
      }
      frame "Validate measurement path" {
        # "Validate the measurement path and set warning if required"
        n130 = Unbundle By Name(w295) -> ("Measurement file/folder path"=w297:path, "LabVIEW Version"=w298:string)
        n131 = call <vilib>:"Is Path and Not Empty.vi"("path"=w297) -> ("Is Path and Not Empty?"=w296:bool)  [unwired: 4 in]
        n132 = case "Is Path and not empty?" shown="True" w296 {
          tunnel: w300 -> [w302 w308]
          tunnel: w297 -> [_ w307]
          tunnel: w298 -> [_ w306]
          tunnel: [w302 w305] -> w299
          tunnel: [w301 w304] -> w292
          tunnel: [_ w303] -> w294
          frame False {
            # "Set warning"
            n133 = call "Warnings.vi"() -> ("Invalid measurement path"=w301:string)  [unwired: 8 in, 7 out]
          }
          frame True {
            # "Validate the path"
            n134 = call "Validate Measurement Path.vi"("Measurement path"=w307, "LabVIEW version"=w306, "error in (no error)"=w308) -> ("Folder?"=w303:bool, "Warning"=w304:string, "error out"=w305:errorcluster)  [unwired: 10 in]
          }
        }
        n135 = Bundle By Name(cluster=w295, "Measurement folder selected?"=w294, "Measurement warning"=w292) -> (w293:T3)
      }
      frame "Validate inputs" {
        # "Validate the project path and measurement path inputs"
        n136 = Unbundle By Name(w322) -> ("Project warning"=w316:string, "Measurement warning"=w321:string, "Next clicked?"=w317:bool, "Project warning"=w315:string, "Measurement warning"=w314:string, "Measurement folder selected?"=w313:bool, "Measurement path changed?"=w312:bool)
        n137 = Empty String/Path?(string/path=w321) -> (empty?=w320:bool)
        n138 = Empty String/Path?(string/path=w316) -> (empty?=w319:bool)
        n139 = And(x=w319, y=w320) -> (x .and. y?=w318:bool)
        n140 = case "Valid inputs?" shown="True" w318 {
          tunnel: w324 -> [w338 w348]
          tunnel: [w333 w344] -> w323
          tunnel: w317 -> [_ w342]
          tunnel: w315 -> [w326 _]
          tunnel: w314 -> [w329 _]
          tunnel: w313 -> [_ w341]
          tunnel: w312 -> [w325 w340]
          tunnel: [w325 w339] -> w309
          frame False {
            # "Set the appropriate warning"
            n141 = call "Edit Warning.vi"("Warning in"=w326) -> ("Warning out"=w328:string)  [unwired: 6 in]
            n142 = call "Edit Warning.vi"("Warning in"=w329) -> ("Warning out"=w327:string)  [unwired: 6 in]
            n143 = Concatenate Strings("Warning:" ("string"), "\n", w328, w327) -> (w331:string)
            n144 = call "Get Warning Position.vi"("Warning"=w331) -> ("Warning position"=w330:i32)  [unwired: 6 in]
            n145 = property on="Warning" class="Bool"(error in=w338, "Visible"=TRUE, "Caption.Text"=w331, "Caption.Top"=w330) -> (error out=w334:errorcluster)  [unwired: 1 in, 1 out]
            n146 = property on="Populate measurements" class="Bool"(error in=w334, "DisabledEnum"=T4."Disabled and Grayed Out" ("Disabled")) -> (error out=w333:errorcluster)  [unwired: 1 in, 1 out]
          }
          frame True {
            # "Check if next is clicked and make the warning invisible"
            n147 = case "Next clicked?" shown="True" w342 {
              tunnel: w348 -> [w350 w355]
              tunnel: [w350 w354] -> w347
              tunnel: w341 -> [_ w353]
              tunnel: w340 -> [w349 w352]
              tunnel: [w349 FALSE] -> w339
              frame False {
                # "Pass"
              }
              frame True {
                # "Populate measurements if folder is selected and List the plug-ins if not"
                n148 = case "Measurement path changed?" shown="True" w352 {
                  tunnel: w355 -> [w361 w368]
                  tunnel: [w360 w367] -> w354
                  tunnel: w353 -> [w356 w365]
                  frame False {
                    # "Measurement folder?"
                    n149 = Select(t=T1."Select measurements" ("Tab Control"), s=w356, f=T1."List Plug-ins" ("Tab Control")) -> (s? t:f=w357:T1)
                    n150 = property on="Tab Control" class="TabCtl (strict)"(error in=w361, "Value"=w357) -> (error out=w360:errorcluster)  [unwired: 1 in, 1 out]
                  }
                  frame True {
                    # "Measurement folder?"
                    n151 = Select(t=string[] ["Populate measurements"] ("States[]"), s=w365, f=string[] ["List plug-ins", "Validate plug-in rename"]) -> (s? t:f=w363:string[])
                    n152 = call "Queue Driver.vi"("States[]"=w363, "error in (no error)"=w368, "Q Operations"=Queue_Operations."Enqueue N") -> ("error out"=w367:errorcluster)  [unwired: 11 in, 1 out]
                  }
                }
              }
            }
            n153 = property on="Warning" class="Bool"(error in=w347, "Visible"=FALSE) -> (error out=w345:errorcluster)  [unwired: 1 in, 1 out]
            n154 = property on="Populate measurements" class="Bool"(error in=w345, "DisabledEnum"=T4."Enabled" ("Disabled")) -> (error out=w344:errorcluster)  [unwired: 1 in, 1 out]
          }
        }
        n155 = Bundle By Name(cluster=w322, "Next clicked?"=FALSE, "Measurement path changed?"=w309) -> (w311:T3)
      }
      frame "/**********FUNCTIONALITY**********/" {
      }
      frame "Populate measurements" {
        w375 = TRUE ("Visible")
        # "Populate the measurements in the Tree and set icon to the items"
        n156 = Unbundle By Name(w388) -> ("Tree Reference"=w382:refnum<vi>, "Measurement file/folder path"=w391:path, "LabVIEW Version"=w389:string)
        n157 = call "Set Cursor Icon.vi"("Cursor icon"=u16 2, "error in (no error)"=w386) -> ("error out"=w385:errorcluster)  [unwired: 13 in]
        n158 = property on="Info" class="Str"(error in=w385, "Visible"=w375, "Text.FontBold"=w375, "Text.Text"="Populating the measurements..." ("Info")) -> (error out=w384:errorcluster)  [unwired: 1 in, 1 out]
        n159 = call "Get Measurements.vi"("Input path"=w391, "LabVIEW version"=w389, "error in (no error)"=w384) -> ("Error?"=w376:string, "VI list"=w378:T10[], "Folder list"=w377:T10[], "error out"=w390:errorcluster)  [unwired: 9 in]
        n160 = Empty String/Path?(string/path=w376) -> (empty?=w379:bool)
        n161 = case "No error occured during get measurements?" shown="True" w379 {
          tunnel: w390 -> [w392 w424]
          tunnel: w388 -> [w399 w423]
          tunnel: [w398 w422] -> w387
          tunnel: w382 -> [w397 w421]
          tunnel: [w395 w420] -> w372
          tunnel: w378 -> [_ w411]
          tunnel: w377 -> [_ w410]
          tunnel: w376 -> [w396 _]
          frame False {
            # "Update the warning"
            n162 = Bundle By Name(cluster=w399, "Tree Reference"=w397, "Measurement warning"=w396) -> (w398:T3)
            n163 = call "Queue Driver.vi"("State"="Validate inputs", "error in (no error)"=w392, "Q Operations"=Queue_Operations."Enqueue") -> ("error out"=w395:errorcluster)  [unwired: 11 in, 1 out]
          }
          frame True {
            w409 = FALSE
            # "Populate the Tree with the measurements"
            n164 = call "Populate Tree.vi"("TreeControl in"=w421, "VI list"=w411, "Folder list"=w410, "error in (no error)"=w424) -> ("TreeControl out"=w418:refnum<vi>, "error out"=w419:errorcluster)  [unwired: 10 in]
            n165 = call "Set Tree Item Icon.vi"("TreeControl in"=w418, "error in (no error)"=w419) -> ("TreeControl out"=w414:refnum<vi>, "Measurement folder Tags"=w412:string[], "Measurement file Tags"=w413:string[], "error out"=w417:errorcluster)  [unwired: 10 in]
            n166 = Empty Array?(array=w413) -> (empty?=w402:bool)
            n167 = Select(t="No Measurement found in the folder" ("Warning"), s=w402, f="Atleast one measurement should be selected" ("Text.Text")) -> (s? t:f=w403:string)
            n168 = property on="Selection warning" class="Str"(error in=w417, "Visible"=TRUE, "Text.Text"=w403) -> (error out=w408:errorcluster)  [unwired: 1 in, 1 out]
            n169 = Select(t=T4."Disabled and Grayed Out" ("Disabled"), s=w402, f=T4."Enabled") -> (s? t:f=w401:T4)
            n170 = Bundle By Name(cluster=w423, "Tree Reference"=w414, "Measurement folder Tags"=w412, "Measurement file Tags"=w413, "Select all"=w409) -> (w422:T3)
            n171 = property on="Select all" class="Bool (strict)"(error in=w408, "Value"=w409, "DisabledEnum"=w401) -> (error out=w415:errorcluster)  [unwired: 1 in, 1 out]
            n172 = property on="Tab Control" class="TabCtl (strict)"(error in=w415, "Value"=T1."Select measurements" ("Tab Control")) -> (error out=w420:errorcluster)  [unwired: 1 in, 1 out]
          }
        }
        n173 = property on="Info" class="Str"(error in=w372, "Visible"=FALSE) -> (error out=w371:errorcluster)  [unwired: 1 in, 1 out]
        n174 = call "Set Cursor Icon.vi"("Cursor icon"=u16 0, "error in (no error)"=w371) -> ("error out"=w381:errorcluster)  [unwired: 13 in]
      }
      frame "Select/Deselect all" {
        # "Update the selection of items in the Tree based on the value of Select all"
        n175 = call "Set Cursor Icon.vi"("Cursor icon"=u16 2, "error in (no error)"=w439) -> ("error out"=w428:errorcluster)  [unwired: 13 in]
        n176 = Unbundle By Name(w431) -> ("Tree Reference"=w432:refnum<vi>, "Measurement folder Tags"=w434:string[], "Measurement file Tags"=w436:string[], "Select all"=w438:bool)
        n177 = Not(x=w438) -> (.not. x?=w440:bool)
        n178 = call "Tree Icons.vi"() -> ("Not Selected"=w442:i32, "Selected"=w443:i32)  [unwired: 6 in]
        n179 = property on="Selection warning" class="Str"(error in=w428, "Text.Text"="Atleast one measurement should be selected", "Visible"=w440) -> (error out=w437:errorcluster)  [unwired: 1 in, 1 out]
        n180 = Select(t=w443, s=w438, f=w442) -> (s? t:f=w435:i32)
        n181 = call "Update Tree Item Icon.vi"("TreeControl in"=w432, "Measurement folder Tags"=w434, "Measurement file Tags"=w436, "Icon"=w435, "error in (no error)"=w437) -> ("TreeControl out"=w429:refnum<vi>, "error out"=w433:errorcluster)  [unwired: 9 in]
        n182 = Bundle By Name(cluster=w431, "Tree Reference"=w429) -> (w430:T3)
        n183 = call "Set Cursor Icon.vi"("Cursor icon"=u16 0, "error in (no error)"=w433) -> ("error out"=w427:errorcluster)  [unwired: 13 in]
      }
      frame "Measurement selection" {
        # "Update the icons of the Tree items based on the selection"
        n184 = call "Set Cursor Icon.vi"("Cursor icon"=u16 2, "error in (no error)"=w464) -> ("error out"=w449:errorcluster)  [unwired: 13 in]
        n185 = Unbundle By Name(w463) -> ("Tree Reference"=w444:refnum<vi>, "Measurement folder Tags"=w454:string[], "Measurement file Tags"=w453:string[], "Selected cell Tag"=w455:string)
        n186 = call "Update Tree Item Selection.vi"("TreeControl in"=w444, "Measurement folder Tags"=w454, "Measurement file Tags"=w453, "Selected cell Tag"=w455, "error in (no error)"=w449) -> ("TreeControl out"=w450:refnum<vi>, "error out"=w460:errorcluster)  [unwired: 9 in]
        n187 = Insert Into Array(array=w454, new element=w453) -> (w456:string[])  [unwired: 1 in]
        n188 = call "Verify Select All.vi"("TreeControl in"=w450, "Measurement Tags"=w456, "error in (no error)"=w460) -> ("TreeControl out"=w452:refnum<vi>, "Select"=w445:bool, "Deselect"=w451:bool, "error out"=w459:errorcluster)  [unwired: 9 in]
        n189 = Bundle By Name(cluster=w463, "Tree Reference"=w452, "Select all"=w445) -> (w462:T3)
        n190 = property on="Select all" class="Bool (strict)"(error in=w459, "Value"=w445) -> (error out=w458:errorcluster)  [unwired: 1 in, 1 out]
        n191 = property on="Selection warning" class="Str"(error in=w458, "Text.Text"="Atleast one measurement should be selected", "Visible"=w451) -> (error out=w461:errorcluster)  [unwired: 1 in, 1 out]
        n192 = call "Set Cursor Icon.vi"("Cursor icon"=u16 0, "error in (no error)"=w461) -> ("error out"=w447:errorcluster)  [unwired: 13 in]
      }
      frame "List plug-ins" {
        # "List the Plug-in names of the selected measurements"
        n193 = Unbundle By Name(w470) -> ("Tree Reference"=w475:refnum<vi>, "Measurement file Tags"=w481:string[], "Measurement folder selected?"=w484:bool, "Measurement file/folder path"=w483:path)
        n194 = call "Set Cursor Icon.vi"("Cursor icon"=u16 2, "error in (no error)"=w485) -> ("error out"=w474:errorcluster)  [unwired: 13 in]
        n195 = case "Measurement Folder?" shown="True" w484 {
          tunnel: w474 -> [w500 w506]
          tunnel: w483 -> [w499 _]
          tunnel: [w498 w503] -> w482
          tunnel: [w496 w502] -> w467
          tunnel: w481 -> [_ w505]
          tunnel: w475 -> [w495 w504]
          tunnel: [w495 w501] -> w468
          frame False {
            # "Get the plug-in name of the selected measurement file"
            n196 = call <vilib>:"Get File Extension.vi"("error in (no error)"=w500, "file"=w499) -> ("error out"=w498:errorcluster, "filename without extension"=w494:string)  [unwired: 5 in, 3 out]
            n197 = Build Array(w494, w494) -> (w497:string[])
            n198 = Build Array(w497) -> (w496:string[][])
          }
          frame True {
            # "Get the plug-in names of all the selected files in the measurement folder"
            n199 = call "Get Selected Measurements.vi"("Tree control in"=w504, "Measurement file Tags"=w505, "error in (no error)"=w506) -> ("Tree control out"=w501:refnum<vi>, "Measurement Plug-ins"=w502:string[][], "error out"=w503:errorcluster)  [unwired: 10 in]
          }
        }
        n200 = Index Array(array=w467, index (col)=0 ("index (row)")) -> (element=w466:string[])  [unwired: 1 in]
        n201 = property on="List of Selected Measurements" class="MCListbox (strict)"(error in=w482, "ItemNames"=w467, "TopLeft"=T5 {"Row"=0, "Column"=0} ("Top Left Visible Cell")) -> (error out=w480:errorcluster)  [unwired: 1 in, 1 out]
        n202 = Bundle By Name(cluster=w470, "Tree Reference"=w468, "Measurement Plug-ins"=w467, "Selected Measurement"=w466) -> (w469:T3)
        n203 = Array Size(array=w467) -> (size(s)=w478:i32[])
        n204 = Index Array(array=w478) -> (element=w477:i32)  [unwired: 1 in]
        n205 = for {
          N: w477 -> [_]
          shift-right: [w491] -> w479
          shift-left: w480 -> [w492]
          i -> [w488]
          # "Set the row size for the occupied rows"
          n206 = Bundle By Name(cluster=T6 {"Row"=0, "Column"=0} ("Active Cell:Active Cell"), "Row"=w488) -> (w490:T6)
          n207 = property on="List of Selected Measurements" class="MCListbox (strict)"(error in=w492, "ActiveCell"=w490, "Height"=u32 18 ("Active Cell:Cell Size:Height")) -> (error out=w491:errorcluster)  [unwired: 1 in, 1 out]
        }
        n208 = property on="Tab Control" class="TabCtl (strict)"(error in=w479, "Value"=T1."List Plug-ins" ("Tab Control")) -> (error out=w487:errorcluster)  [unwired: 1 in, 1 out]
        n209 = call "Set Cursor Icon.vi"("Cursor icon"=u16 0, "error in (no error)"=w487) -> ("error out"=w472:errorcluster)  [unwired: 13 in]
      }
      frame "Update plugin name" {
        n210 = property on="List of Selected Measurements" class="MCListbox (strict)"(error in=w511) -> (error out=w510:errorcluster, "ItemNames"=w507:string[][])  [unwired: 1 in, 1 out]
        n211 = Bundle By Name(cluster=w509, "Measurement Plug-ins"=w507) -> (w508:T3)
      }
      frame "Validate plug-in rename" {
        # "Validate the name of the Plug-in after rename"
        n212 = call "Set Cursor Icon.vi"("Cursor icon"=u16 2, "error in (no error)"=w547) -> ("error out"=w539:errorcluster)  [unwired: 13 in]
        n213 = property on="List of Selected Measurements" class="MCListbox (strict)"(error in=w539) -> (error out=w531:errorcluster, "ItemNames"=w545:string[][])  [unwired: 1 in, 1 out]
        n214 = Unbundle By Name(w543) -> ("Measurement Plug-ins"=w541:string[][], "Project path"=w529:path)
        n215 = Index Array(array=w545, index (col)=1 ("disabled index (col)")) -> (element=w514:string[])  [unwired: 1 in]
        n216 = call "Get Libraries in Project.vi"("Project path"=w529, "error in (no error)"=w531) -> ("Project exists?"=w528:bool, "Library names"=w527:string[], "error out"=w530:errorcluster)  [unwired: 11 in]
        n217 = Index Array(array=w541, index (col)=1 ("disabled index (col)")) -> (element=w513:string[])  [unwired: 1 in]
        n218 = for {
          shift-right: [w554] -> w524
          shift-left: w530 -> [w555]
          tunnel: w514 -> [w551] mode=indexing
          tunnel: w528 -> [w553]
          tunnel: w527 -> [w552]
          tunnel: [w549] -> w515 mode=indexing
          tunnel: w513 -> [w550] mode=indexing
          tunnel: [w548] -> w512 mode=indexing
          # "Validate the plug-in names"
          n219 = call "Validate Plugin Name.vi"("Project exists?"=w553, "Library names"=w552, "Plug-in name"=w551, "error in (no error)"=w555) -> ("Valid Name?"=w549:bool, "error out"=w554:errorcluster)  [unwired: 10 in]
          n220 = Swap Values(12:w550, 13:w549, 14:w551) -> (1:w548:string)  [unwired: 1 out]
        }
        n221 = call "Set Plug-in Name Warning.vi"("Valid Name?"=w515, "Validated names"=w512, "error in (no error)"=w524) -> ("Warning?"=w525:bool, "error out"=w523:errorcluster)  [unwired: 11 in]
        n222 = Replace Array Subset(array=w541, new element=w512, index (col)=1 ("disabled index (col)")) -> (w516:string[][])  [unwired: 1 in]
        n223 = property on="Plug-in warning" class="Str"(error in=w523, "Visible"=w525) -> (error out=w535:errorcluster)  [unwired: 1 in, 1 out]
        n224 = Swap Values(12:u32 250 ("Size:Height"), 13:w525, 14:210 ("x")) -> (1:w526:u32)  [unwired: 1 out]
        n225 = Bundle By Name(cluster=w543, "Measurement Plug-ins"=w516) -> (w542:T3)
        n226 = property on="List of Selected Measurements" class="MCListbox (strict)"(error in=w535, "ItemNames"=w516, "Height"=w526) -> (error out=w532:errorcluster)  [unwired: 1 in, 1 out]
        n227 = Not(x=w525) -> (.not. x?=w520:bool)
        n228 = property on="Plug-in info" class="Str"(error in=w532, "Visible"=w520) -> (error out=w522:errorcluster)  [unwired: 1 in, 1 out]
        n229 = Select(t=T4."Enabled", s=w520, f=T4."Disabled and Grayed Out" ("Disabled")) -> (s? t:f=w517:T4)
        n230 = property on="Start Migration" class="Bool"(error in=w522, "DisabledEnum"=w517) -> (error out=w521:errorcluster)  [unwired: 1 in, 1 out]
        n231 = call "Set Cursor Icon.vi"("Cursor icon"=u16 0, "error in (no error)"=w521) -> ("error out"=w537:errorcluster)  [unwired: 13 in]
      }
      frame "/**********MULTIPLE MIGRATION**********/" {
      }
      frame "Update Measurement Paths" {
        w571 = 70  # Remaining Progress
        # "Update the measurement file paths for measurement folder"
        n232 = property on="Progress" class="Slide (strict)"(error in=w564, "Value"=5 ("Progress"), "Caption.Text"="Getting paths...") -> (error out=w572:errorcluster)  [unwired: 1 in, 1 out]
        n233 = Unbundle By Name(w577) -> ("Migration Status"=w567:string[][], "Measurement file/folder path"=w580:path, "Measurement Plug-ins"=w579:string[][], "Measurement folder selected?"=w578:bool, "Selected Measurement"=w558:string[])  [unwired: 1 out]
        n234 = property on="Measurement Count" class="Slide (strict)"(error in=w572, "Value"=0 ("Measurement Count"), "Caption.Text"="Updating Measurement Paths") -> (error out=w568:errorcluster)  [unwired: 1 in, 1 out]
        n235 = call "Get Measurement Paths.vi"("Measurement Path"=w580, "Measurement Plug-ins"=w579, "Measurement folder selected?"=w578, "error in"=w568) -> ("Measurement Path Array"=w575:path[], "error out"=w560:errorcluster)  [unwired: 10 in]
        n236 = Insert Into Array(array=w567, index (col)=0 ("disabled index (col)"), new element=w558) -> (w565:string[][])  [unwired: 1 in]
        n237 = Array Size(array=w575) -> (size(s)=w570:i32)
        n238 = Quotient & Remainder(x=w571, y=w570) -> (floor(x/y)=w569:i32)  [unwired: 1 out]
        n239 = Bundle By Name(cluster=w577, "Migration Status"=w565, "Measurement File Paths"=w575, "Plugin Migration Value"=w570, "Progress per measurement"=w569) -> (w576:T3)
        n240 = property on="Progress" class="Slide (strict)"(error in=w560, "Value"=15 ("Progress")) -> (error out=w559:errorcluster)  [unwired: 1 in, 1 out]
      }
      frame "Create Project" {
        # "Check if project exists and creates a new project if not present."
        n241 = property on="Progress" class="Slide (strict)"(error in=w584, "Value"=10 ("Progress"), "Caption.Text"="Checking for project...") -> (error out=w585:errorcluster)  [unwired: 1 in, 1 out]
        n242 = property on="Measurement Count" class="Slide (strict)"(error in=w585, "Value"=10 ("Measurement Count"), "Caption.Text"="Creating project if not exist") -> (error out=w588:errorcluster)  [unwired: 1 in, 1 out]
        n243 = Unbundle By Name(w592) -> ("Project path"=w591:path)
        n244 = call "Create and Save Project.vi"("Project Path"=w591, "error in (no error)"=w588) -> ("error out"=w582:errorcluster)  [unwired: 13 in]
        n245 = property on="Progress" class="Slide (strict)"(error in=w582, "Value"=15 ("Progress")) -> (error out=w581:errorcluster)  [unwired: 1 in, 1 out]
      }
      frame "Migrate measurements" {
        # "Migrate multiple measurements along with their shared dependencies"
        n246 = property on="Progress" class="Slide (strict)"(error in=w594, "Value"=0 ("Progress")) -> (error out=w595:errorcluster)  [unwired: 1 in, 1 out]
        n247 = Unbundle By Name(w605) -> ("Project path"=w609:path, "Measurement File Paths"=w607:path[], "Measurement Plug-ins"=w610:string[][])
        n248 = property on="Measurement Count" class="Slide (strict)"(error in=w595, "Value"=20 ("Measurement Count"), "Caption.Text"="Migrating measurement(s)") -> (error out=w600:errorcluster)  [unwired: 1 in, 1 out]
        n249 = Index Array(array=w610, index (col)=1 ("disabled index (col)")) -> (element=w608:string[])  [unwired: 1 in]
        n250 = control-ref of="Progress"() -> (w593:refnum<vi>)
        n251 = call "Migrate Dependencies.vi"("Project path"=w609, "Measurement paths"=w607, "Plug-in names"=w608, "Progress"=w593, "error in"=w600) -> ("Instrument containing subVIs"=w604:path[][], "error out"=w598:errorcluster)  [unwired: 9 in]
        n252 = Bundle By Name(cluster=w605, "Instrument containing subVIs"=w604, "Measurement Progress"=30) -> (w606:T3)
        n253 = property on="Measurement Count" class="Slide (strict)"(error in=w598, "Value"=30 ("Measurement Count")) -> (error out=w597:errorcluster)  [unwired: 1 in, 1 out]
      }
      frame "Enqueue Migration Steps" {
        # "Enqueue the set of states for measurement migration"
        n254 = Unbundle By Name(w616) -> ("Plugin Migration Value"=w615:i32)
        n255 = Greater Than 0?(x=w615) -> (x > 0?=w614:bool)
        n256 = case shown="True" w614 {
          tunnel: w613 -> [w619 w626]
          tunnel: [w621 w625] -> w612
          frame False {
            # "Enqueue next step if all measurements are migrated"
            n257 = property on="Measurement Count" class="Slide (strict)"(error in=w619, "Value"=100 ("Progress")) -> (error out=w620:errorcluster)  [unwired: 1 in, 1 out]
            n258 = call "Queue Driver.vi"("States[]"=string[] ["Save Project", "Show Next Steps"], "error in (no error)"=w620, "Q Operations"=Queue_Operations."Enqueue N") -> ("error out"=w621:errorcluster)  [unwired: 11 in, 1 out]
          }
          frame True {
            # "Enqueue, if there are measurements yet to migrate"
            n259 = call "Queue Driver.vi"("States[]"=string[] ["Set Values in Dict", "Create Plugin Template", "Get Driver List", "Edit Measurement Configuration", "Edit Measurement Results", "Edit Measurement Connector Pane", "Create Wrapper", "Deserialize Cluster Data", "Add Measurement Plugin APIs", "Disable Initialize APIs", "Edit Type Specialization", "Add UI Elements", "Flatten the Clusters", "Handling Default Value", "Update Migration Count"], "error in (no error)"=w626, "Q Operations"=Queue_Operations."Enqueue N") -> ("error out"=w625:errorcluster)  [unwired: 11 in, 1 out]
          }
        }
      }
      frame "Set Values in Dict" {
        # "Measurement Status Message: Migrating 1 of N measurement(s)"
        # "Set values to the Dictionary APIs"
        n260 = Unbundle By Name(w649) -> ("Project path"=w643:path, "Instrument containing subVIs"=w639:path[][], "Measurement Plug-ins"=w648:string[][], "Migration Count"=w627:i32, "Measurement File Paths"=w636:path[])
        n261 = property on="Progress" class="Slide (strict)"(error in=w630, "Value"=0 ("Progress")) -> (error out=w635:errorcluster)  [unwired: 1 in, 1 out]
        n262 = Array Size(array=w636) -> (size(s)=w628:i32)
        n263 = Increment(x=w627) -> (x+1=w632:i32)
        n264 = Format Into String(format string="Migrating %d of %d measurement(s)", error in=w635, w632, w628) -> (resulting string=w633:string, error out=w634:errorcluster)  [unwired: 1 in]
        n265 = property on="Measurement Count" class="Slide (strict)"(error in=w634, "Caption.Text"=w633) -> (error out=w637:errorcluster)  [unwired: 1 in, 1 out]
        n266 = Index Array(array=w636, index=w627) -> (element=w646:path)
        n267 = call "Set Code Module Path.vi"("CodeModule Path"=w646, "error in (no error)"=w637) -> ("error out"=w645:errorcluster)  [unwired: 13 in]
        n268 = Index Array(array=w648, index (row)=w627, index (col)=1 ("disabled index (col)")) -> (element=w644:string)
        n269 = Index Array(array=w639, index (row)=w627) -> (element=w642:path[])  [unwired: 1 in]
        n270 = call "Set Measurement Name.vi"("Name"=w644, "error in (no error)"=w645) -> ("error out"=w641:errorcluster)  [unwired: 13 in]
        n271 = call "Set Instrument VI Paths.vi"("error in (no error)"=w641, "VI Paths[]"=w642) -> ("error out"=w640:errorcluster)  [unwired: 9 in]
        n272 = call "Set Project Path.vi"("Project Path"=w643, "error in (no error)"=w640) -> ("error out"=w629:errorcluster)  [unwired: 13 in]
      }
      frame "Create Plugin Template" {
        # "Create Measurement Plugin Template"
        n273 = property on="Progress" class="Slide (strict)"(error in=w664, "Value"=1 ("Progress"), "Caption.Text"="Creating G Plugin...") -> (error out=w661:errorcluster)  [unwired: 1 in, 1 out]
        n274 = call "Copy Gplugin datafile.vi"("error in (no error)"=w661) -> ("G PLugin File Path"=w652:path, "error out"=w662:errorcluster)  [unwired: 13 in]
        n275 = call "Create PPL.vi"("error in (no error)"=w662) -> ("error out"=w660:errorcluster)  [unwired: 14 in]
        n276 = call "Copy plugin Sdk template.vi"("error in (no error)"=w660) -> ("error out"=w659:errorcluster)  [unwired: 14 in]
        n277 = call "Hide the SessionId.vi"("error in (no error)"=w659) -> ("error out"=w658:errorcluster)  [unwired: 14 in]
        n278 = call "Get Library Name.vi"("error in (no error)"=w658) -> ("VI Path"=w654:path, "Lib Name"=w656:string, "VI Name"=w655:string, "error out"=w657:errorcluster)  [unwired: 11 in]
        n279 = call "Edit gplugin data file.vi"("Path"=w652, "Lib Name"=w656, "VI Name"=w655, "error in (no error)"=w657) -> ("error out"=w650:errorcluster)  [unwired: 11 in]
        n280 = in-place {
          in-place-border: w654 -> [w669]
          in-place-border: w652 -> [w666]
          n281 = in-place-cluster #2(w653) -> ("G plugin Path"=w671:path[], "Plugin data file"=w670:path[])
          n282 = Insert Into Array(array=w671, new element=w669) -> (w668:path[])  [unwired: 1 in]
          n283 = Insert Into Array(array=w670, new element=w666) -> (w667:path[])  [unwired: 1 in]
          n284 = in-place-cluster #2("G plugin Path"=w668, "Plugin data file"=w667) -> (w651:T3)
        }
      }
      frame "Save Project" {
        # "Saving the project and libraries"
        n285 = property on="Progress" class="Slide (strict)"(error in=w673, "Value"=15 ("Progress"), "Caption.Text"="Saving the project files...") -> (error out=w675:errorcluster)  [unwired: 1 in, 1 out]
        n286 = call "Save Projects and Libraries.vi"("error in (no error)"=w675) -> ("error out"=w674:errorcluster)  [unwired: 10 in]
      }
      frame "Update Migration Count" {
        # "Updating the migration count and migration status"
        n287 = in-place {
          in-place-border: [w686] -> w680
          n288 = in-place-cluster #3(w685) -> ("Plugin Migration Value"=w698:i32, "Migration Count"=w689:i32, "Measurement Progress"=w696:i32, "Progress per measurement"=w695:i32, "Migration Status"=w692:string[][])
          n289 = Index Array(array=w692, index (col)=1 ("disabled index (col)")) -> (element=w690:string[])  [unwired: 1 in]
          n290 = Insert Into Array(array=w690, index=w689, new element="Success") -> (w687:string[])
          n291 = Insert Into Array(array=w692, index (col)=1 ("disabled index (col)"), new element=w687) -> (w694:string[][])  [unwired: 1 in]
          n292 = Increment(x=w689) -> (x+1=w699:i32)
          n293 = Add(x=w696, y=w695) -> (x+y=w686:i32)
          n294 = Decrement(x=w698) -> (x-1=w697:i32)
          n295 = in-place-cluster #3("Plugin Migration Value"=w697, "Migration Count"=w699, "Measurement Progress"=w686, "Progress per measurement"=w695, "Migration Status"=w694) -> (w684:T3)
        }
        n296 = property on="Measurement Count" class="Slide (strict)"(error in=w679, "Value"=w680) -> (error out=w678:errorcluster)  [unwired: 1 in, 1 out]
        n297 = call "Queue Driver.vi"("State"="Enqueue Migration Steps", "error in (no error)"=w678, "Q Operations"=Queue_Operations."Enqueue") -> ("error out"=w683:errorcluster)  [unwired: 11 in, 1 out]
      }
      frame "Update count on Fail" {
        # "Updating the migration count and migration status"
        n298 = in-place {
          in-place-border: [w708] -> w702
          n299 = in-place-cluster #4(w707) -> ("Plugin Migration Value"=w720:i32, "Migration Count"=w711:i32, "Measurement Progress"=w718:i32, "Progress per measurement"=w717:i32, "Migration Status"=w714:string[][])
          n300 = Index Array(array=w714, index (col)=1 ("disabled index (col)")) -> (element=w712:string[])  [unwired: 1 in]
          n301 = Insert Into Array(array=w712, index=w711, new element="Fail") -> (w709:string[])
          n302 = Insert Into Array(array=w714, index (col)=1 ("disabled index (col)"), new element=w709) -> (w716:string[][])  [unwired: 1 in]
          n303 = Increment(x=w711) -> (x+1=w721:i32)
          n304 = Add(x=w718, y=w717) -> (x+y=w708:i32)
          n305 = Decrement(x=w720) -> (x-1=w719:i32)
          n306 = in-place-cluster #4("Plugin Migration Value"=w719, "Migration Count"=w721, "Measurement Progress"=w708, "Progress per measurement"=w717, "Migration Status"=w716) -> (w706:T3)
        }
        n307 = property on="Measurement Count" class="Slide (strict)"(error in=w701, "Value"=w702) -> (error out=w700:errorcluster)  [unwired: 1 in, 1 out]
        n308 = call "Queue Driver.vi"("State"="Enqueue Migration Steps", "error in (no error)"=w700, "Q Operations"=Queue_Operations."Enqueue") -> ("error out"=w705:errorcluster)  [unwired: 11 in, 1 out]
      }
      frame "/**********NEXT STEPS POST MIGRATION**********/" {
      }
      frame "Show Next Steps" {
        # "To change unwanted loading symbol"
        # "Showing the migration status"
        n309 = in-place {
          in-place-border: [w747] -> w731
          n310 = in-place-cluster #5(w739) -> ("Migration Status"=w748:string[][])
          n311 = Index Array(array=w748, index (col) #1=0 ("disabled index (col)"), index (col) #2=1 ("index (col)")) -> (element #1=w751:string[], element #2=w749:string[])  [unwired: 2 in]
          n312 = for {
            tunnel: w751 -> [_] mode=indexing
            tunnel: w749 -> [w758]
            shift-right: [w753] -> w747
            shift-left: w748 -> [w756]
            i -> [w755]
            n313 = Index Array(array=w758, index=w755) -> (element=w757:string)
            n314 = Empty String/Path?(string/path=w757) -> (empty?=w754:bool)
            n315 = case shown="True" w754 {
              tunnel: w756 -> [w759 w766]
              tunnel: w755 -> [_ w763]
              tunnel: [w759 w767] -> w753
              frame False {
              }
              frame True {
                # "Insert 'Fail' for empty status"
                n316 = Index Array(array=w766, index (col)=1 ("disabled index (col)")) -> (element=w764:string[])  [unwired: 1 in]
                n317 = Insert Into Array(array=w764, index=w763, new element="Fail" ("new element/subarray")) -> (w761:string[])
                n318 = Insert Into Array(array=w766, index (col)=1 ("disabled index (col)"), new element=w761) -> (w767:string[][])  [unwired: 1 in]
              }
            }
          }
          n319 = in-place-cluster #5("Migration Status"=w747) -> (w738:T3)
        }
        n320 = property on="Tab Control" class="TabCtl (strict)"(error in=w734, "Value"=T1."Status" ("Tab Control")) -> (error out=w736:errorcluster)  [unwired: 1 in, 1 out]
        n321 = property on="Migration Status" class="MCListbox (strict)"(error in=w736, "Allow Editing Cells"=FALSE) -> (error out=w735:errorcluster)  [unwired: 1 in, 1 out]
        n322 = property on="Migration Status" class="MCListbox (strict)"(error in=w735, "ItemNames"=w731) -> (error out=w726:errorcluster)  [unwired: 1 in, 1 out]
        n323 = Index Array(array=w731, index (col)=1 ("disabled index (col)")) -> (element=w729:string[])  [unwired: 1 in]
        n324 = Equal?(x=w729, y="Fail" ("new element/subarray")) -> (x = y?=w727:bool[])
        n325 = And Array Elements(Boolean array=w727) -> (logical AND=w724:bool)
        n326 = case "All the measurements failed?" shown="True" w724 {
          tunnel: w726 -> [w742 w746]
          tunnel: [w743 w745] -> w725
          frame False {
            n327 = property on="Review" class="Bool"(error in=w742, "BoolText.Text"="Review Plug-ins" ("Boolean Text.Text")) -> (error out=w743:errorcluster)  [unwired: 1 in, 1 out]
          }
          frame True {
            # "Change Bool Text to Start next migration"
            n328 = property on="Review" class="Bool"(error in=w746, "BoolText.Text"="Start Next Migration" ("Boolean Text.Text")) -> (error out=w745:errorcluster)  [unwired: 1 in, 1 out]
          }
        }
        n329 = call "Set Cursor Icon.vi"("Cursor icon"=u16 0, "error in (no error)"=w725) -> ("error out"=w733:errorcluster)  [unwired: 13 in]
      }
      frame "Show Links" {
        # "Showing links for the migrated measurements"
        n330 = Unbundle By Name(w776) -> ("Migration Status"=w778:string[][])
        n331 = for {
          tunnel: w778 -> [w785] mode=indexing
          tunnel: [w779] -> w773 mode=indexing if=w782
          # "Populating combo box with successfully migrated plugin names"
          n332 = Index Array(array=w785, index #1=0 ("index"), index #2=1 ("index")) -> (element #1=w779:string, element #2=w780:string)
          n333 = Equal?(x=w780, y="Success") -> (x = y?=w782:bool)
        }
        n334 = Index Array(array=w773, index=0) -> (element=w770:string)
        n335 = property on="Select Plug-in" class="CmbBox"(error in=w777, "Strings[]"=w773, "Value"=w770) -> (error out=w771:errorcluster)  [unwired: 1 in, 1 out]
        n336 = Bundle By Name(cluster=w776, "Index"=0) -> (w769:T3)
        n337 = property on="Tab Control" class="TabCtl (strict)"(error in=w771, "Value"=T1."Links" ("Tab Control")) -> (error out=w774:errorcluster)  [unwired: 1 in, 1 out]
      }
      frame "/**********ERROR**********/" {
      }
      frame "Error" {
        # "Handle the error and alert user"
        n338 = call <vilib>:"Clear Errors.vi"("error in (no error)"=w795) -> ("error out"=w796:errorcluster)  [unwired: 5 in, 1 out]
        n339 = Equal?(x=string[] ["Set Values in Dict", "Create Plugin Template", "Get Driver List", "Edit Measurement Configuration", "Edit Measurement Results", "Edit Measurement Connector Pane", "Create Wrapper", "Deserialize Cluster Data", "Add Measurement Plugin APIs", "Disable Initialize APIs", "Edit Type Specialization", "Add UI Elements", "Flatten the Clusters", "Handling Default Value", "Update Migration Count"] ("States[]"), y=w788) -> (x = y?=w790:bool[])
        n340 = call "Queue Driver.vi"("error in (no error)"=w796, "Q Operations"=Queue_Operations."Flush") -> ("error out"=w793:errorcluster)  [unwired: 12 in, 1 out]
        n341 = Or Array Elements(Boolean array=w790) -> (logical OR=w789:bool)
        n342 = case shown="False" w789 {
          tunnel: w793 -> [w803 w815]
          tunnel: [w802 w813] -> w792
          tunnel: w788 -> [w801 _]
          frame False {
            # "If error occurs in other steps"
            n343 = Equal?(x=string[] ["Update Measurement Paths", "Create Project", "Migrate measurements"] ("States[]"), y=w801) -> (x = y?=w799:bool[])
            n344 = Or Array Elements(Boolean array=w799) -> (logical OR=w798:bool)
            n345 = case "Error in Migration?" shown="False" w798 {
              tunnel: w803 -> [w807 w810]
              tunnel: [w806 w809] -> w802
              frame False {
                # "Restart Migration tool"
                n346 = call "Queue Driver.vi"("States[]"=string[] ["Reinitialize", "Initialize UI", "Populate project path"], "error in (no error)"=w807, "Q Operations"=Queue_Operations."Enqueue N") -> ("error out"=w806:errorcluster)  [unwired: 11 in, 1 out]
              }
              frame True {
                # "Show Next steps"
                n347 = call "Queue Driver.vi"("State"="Show Next Steps", "error in (no error)"=w810, "Q Operations"=Queue_Operations."Enqueue") -> ("error out"=w809:errorcluster)  [unwired: 11 in, 1 out]
              }
            }
          }
          frame True {
            # "If error occurs during measurement migration"
            n348 = call "Queue Driver.vi"("State"="Update count on Fail", "error in (no error)"=w815, "Q Operations"=Queue_Operations."Enqueue") -> ("error out"=w813:errorcluster)  [unwired: 11 in, 1 out]
          }
        }
      }
      frame "/**********EXIT**********/" {
      }
      frame "Exit" {
        # "Flush the queue elements and stop execution"
        n349 = call "Queue Driver.vi"("error in (no error)"=w828, "Q Operations"=Queue_Operations."Flush") -> ("error out"=w822:errorcluster)  [unwired: 12 in, 1 out]
        n350 = call "Queue Driver.vi"("error in (no error)"=w822, "Q Operations"=Queue_Operations."Release") -> ("error out"=w821:errorcluster)  [unwired: 12 in, 1 out]
        n351 = Unbundle By Name(w826) -> ("Tree Reference"=w825:refnum<vi>)
        n352 = Close Reference(reference=w825, error in (no error)=w821) -> (error out=w819:errorcluster)
        n353 = call "Dictionary.vi"("error in (no error)"=w819, "Dict States"=Dictionary_States."Delete All") -> ("error out"=w818:errorcluster)  [unwired: 12 in, 1 out]
      }
    }
  }
  n354 = invoke class="VI" method="FP.Close"(error in=w6) -> (error out=→"error out":errorcluster)  [unwired: 2 in, 2 out]
